vi "FT10_Dialog Hardware Connection Failure.vi"(9 "Simulation?":bool, 10 "Connected?":bool, 11 "Hardware":string) -> ()   [LabVIEW 2015]
doc: "Notify user with dialog if hardware fails to connect."
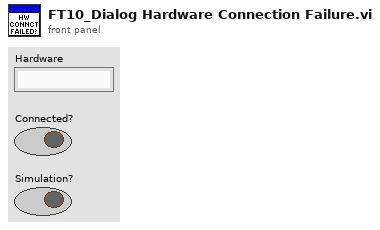
[diagram p1: front panel]
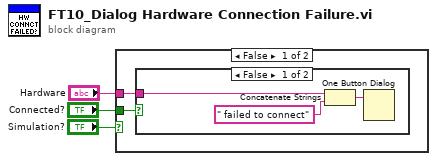
[diagram p0: block diagram]
diagram:
  n1 = case shown="False" "Simulation?" {
    tunnel: "Connected?" -> [w5 _]
    tunnel: "Hardware" -> [w4 _]
    frame False {
      n2 = case shown="False" w5 {
        tunnel: w4 -> [w6 _]
        frame False {
          n3 = Concatenate Strings(w6, " failed to connect" ("message")) -> (w7:string)
          n4 = One Button Dialog(message=w7) -> ()  [unwired: 1 in, 1 out]
        }
        frame True {
        }
      }
    }
    frame True {
    }
  }
